vi "Format to string.vi"(8 "error in (no error)":errorcluster, 11 "address":refnum<class "MacOS Network Address.lvclass">) -> (0 "error out":errorcluster, 2 "address string":string, 3 "address out":refnum<class "MacOS Network Address.lvclass">)   [LabVIEW 2020, in "NI_WFCN.lvlib" / "MacOS Network Address.lvclass"]
doc: "Returns a human-readable string representation of this address."
uses:
  <vilib>/net/WFCN/Addressing/MacOS Network Address/MacOS Network Address.lvclass
  <vilib>/net/WFCN/Addressing/MacOS Network Address/MacOS Network Address.lvclass/MacOS Network Address.ctl
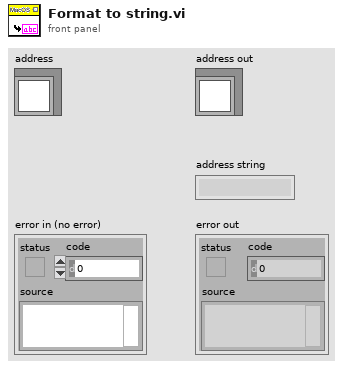
[diagram p1: front panel]
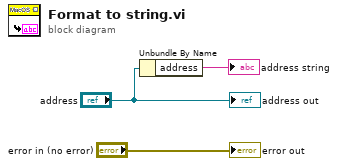
[diagram p0: block diagram]
diagram:
  n1 = Unbundle By Name("address") -> ("address"=→"address string":string)
  "error out" <- "error in (no error)"
  "address out" <- "address"
